vi "Single AIN with config.vi"() -> (0 "error out":errorcluster)   [LabVIEW 2009]
panel:
  out "Voltage":dbl format="%.9f"
  in  "Channel Name":string="AIN0"
  in  "Config Values":dbl[](array[numeric])=[199.0, 10.0, 0.0, 0.0] format="%.2f"
  out "Error String":string
  out "ConnectionType Out":i32
  out "DeviceType Out":i32
  in  "Identifier":string="LJM_idANY"
  in  "ConnectionType":string="LJM_ctANY"
  in  "DeviceType":string="LJM_dtANY"
  in  "Config NumFrames":i32=4
  in  "Config Names":string[](array[string])=["AIN0_NEGATIVE_CH", "AIN0_RANGE", "AIN0_RESOLUTION_INDEX", "AIN0_EF_TYPE"]
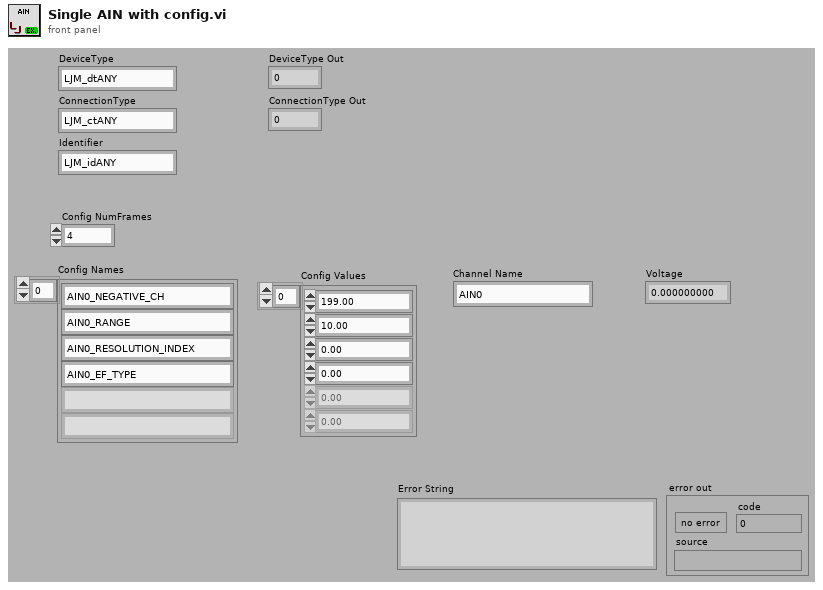
[diagram p1: front panel]
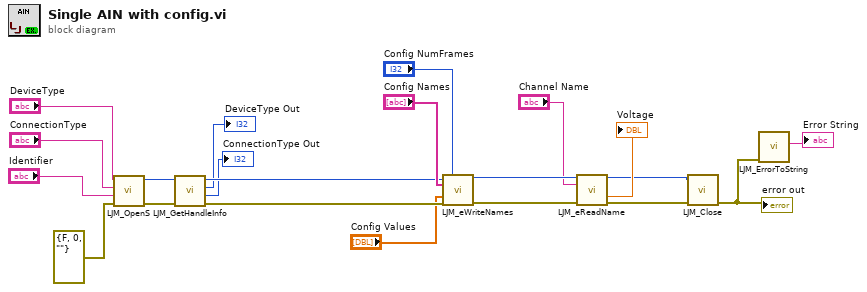
[diagram p0: block diagram]
diagram:
  n1 = call <vilib>:"LJM_OpenS.vi"("error in"=errorcluster {"status"=FALSE, "code"=0, "source"=""} ("error in (no error)"), "Identifier"="Identifier", "ConnectionType"="ConnectionType", "DeviceType"="DeviceType") -> ("error out"=w18:errorcluster, "Handle"=w16:i32)  [unwired: 6 in]
  n2 = call <vilib>:"LJM_GetHandleInfo.vi"("error in"=w18, "Handle In"=w16) -> ("error out"=w17:errorcluster, "ConnectionType"=→"ConnectionType Out":i32, "DeviceType"=→"DeviceType Out":i32, "Handle Out"=w15:i32)  [unwired: 2 in, 4 out]
  n3 = call <vilib>:"LJM_eWriteNames.vi"("Handle In"=w15, "NumFrames"="Config NumFrames", "aNames"="Config Names", "aValuesIn"="Config Values", "error in"=w17) -> ("Handle Out"=w5:i32, "error out"=w6:errorcluster)  [unwired: 8 in, 1 out]
  n4 = call <vilib>:"LJM_eReadName.vi"("Handle In"=w5, "Name"="Channel Name", "error in"=w6) -> ("Handle Out"=w1:i32, "Value"=→"Voltage":dbl, "error out"=w4:errorcluster)  [unwired: 10 in]
  n5 = call <vilib>:"LJM_Close.vi"("error in"=w4, "Handle"=w1) -> ("error out"=w9:errorcluster)  [unwired: 9 in]
  "error out" <- w9
  n6 = call <vilib>:"LJM_ErrorToString.vi"("error in"=w9) -> ("String"=→"Error String":string)  [unwired: 10 in]
